vi "Load Obj File.vi"(5 "Load Material Textures (Default: True)":bool=TRUE, 6 "Material Search Folder (Default: <Not A Path> - Use Model Path Folder)":path=path "", 7 "Force Regenerate Normals (Defaut: False)":bool, 8 "error in (no error)":errorcluster, 11 "Object Model Path":path) -> (0 "error out":errorcluster, 3 "Objects":refnum<vi>[](array[refnum]), 4 "Bounding Box":T1)   [LabVIEW 2020, in "g_ar_toolkit.ar.lvlib"]
uses:
  g_ar_toolkit.ar.lvlib
  Model Bounding Box.ctl
  g_ar_toolkit.common/Object Point (Float).ctl
  Vertex Descriptor.ctl
  <vilib>/Utility/miscctls.llb/LV3DPointTypeDef.ctl
  <vilib>/picture/3D Picture Control/Geometries/Create Mesh.vi
  <vilib>/picture/3D Picture Control/Object/Create Object.vi
  <vilib>/picture/3D Picture Control/Object/Create Object (drawable).vi
  <vilib>/picture/3D Picture Control/Object/Set Material.vi
  <vilib>/Utility/libraryn.llb/Get File Extension.vi
  <vilib>/picture/jpeg.llb/Read JPEG File.vi
  <vilib>/picture/3D Picture Control/Helpers/Apply Texture.vi
  <vilib>/picture/3D Picture Control/Helpers/Apply Texture (no reference).vi
  <vilib>/picture/png.llb/Read PNG File.vi
  <vilib>/picture/bmp.llb/Read BMP File.vi
  bin/g_ar_toolkit.1.32.dll
  g_ar_toolkit.common/g_ar_toolkit.common.lvlib
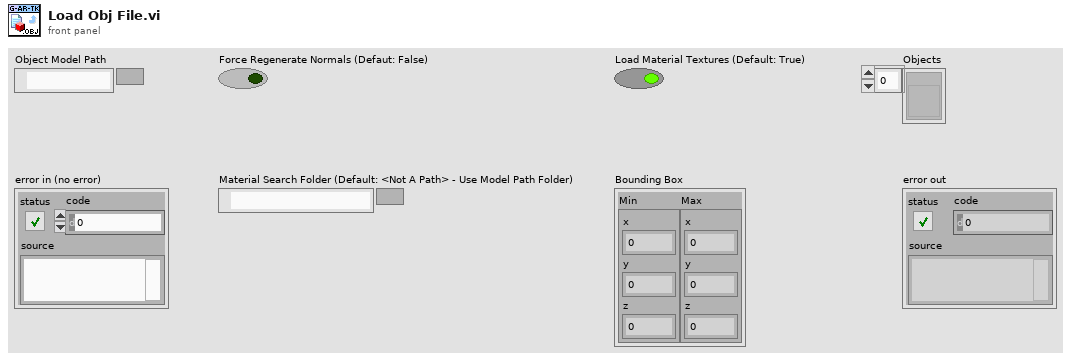
[diagram p1: front panel]
types:
  T1 = typedef "g_ar_toolkit.ar.lvlib/Model Bounding Box.ctl" = cluster{"Min":T2, "Max":T2}
  T2 = typedef "g_ar_toolkit.common.lvlib/Object Point (Float).ctl" = cluster{"x":dbl, "y":dbl, "z":dbl}
  T3 = typedef "g_ar_toolkit.ar.lvlib/Vertex Descriptor.ctl" = cluster{"Vertex":T4, "Normal":T4, "Colour":cluster{"R":sgl, "G":sgl, "B":sgl}, "Texture Coord":cluster{"S":sgl, "T":sgl}}
  T4 = typedef "LV3DPointTypeDef.ctl" = cluster{"X":sgl, "Y":sgl, "Z":sgl}
  T5 = cluster{"Name":string, "Shininess":sgl, "Ambient":cluster{"Red":sgl, "Green":sgl, "Blue":sgl}, "Specular":cluster{"Red":sgl, "Green":sgl, "Blue":sgl}, "Emission":cluster{"Red":sgl, "Green":sgl, "Blue":sgl}, "Diffuse":cluster{"Red":sgl, "Green":sgl, "Blue":sgl}, "texture-name":string}[]
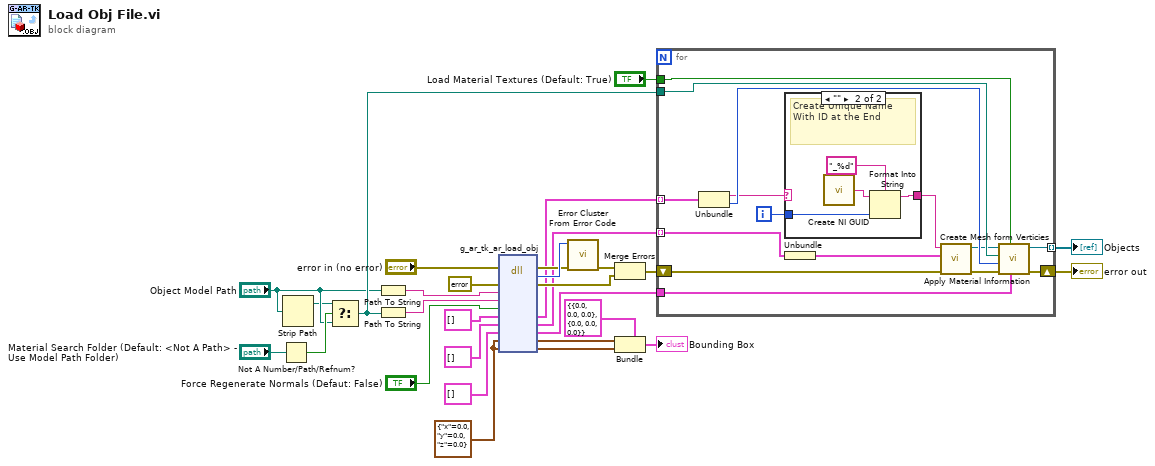
[diagram p0: block diagram]
diagram:
  w20 = T2 {"x"=0.0, "y"=0.0, "z"=0.0} ("Object Point")
  n1 = Not A Number/Path/Refnum?(number/path/refnum="Material Search Folder (Default: <Not A Path> - Use Model Path Folder)") -> (NaN/Path/Refnum?=w4:bool)
  n2 = Strip Path(path="Object Model Path") -> (stripped path=w1:path)  [unwired: 1 out]
  n3 = Select(t=w1, s=w4, f="Object Model Path") -> (s? t:f=w3:path)
  n4 = Path To String(path="Object Model Path") -> (string=w19:string)
  n5 = Path To String(path=w3) -> (string=w18:string)
  n6 = dll-call lib="C:/serenial/libraries/g-augmented-reality-toolkit/LabVIEW/bin/g_ar_toolkit.1.*.*" fn="g_ar_tk_ar_load_obj" ("g_ar_toolkit.*.*:g_ar_tk_image_copy")(error in="error in (no error)", "error_cluster"=errorcluster {"status"=FALSE, "code"=0, "source"=""} ("error constant"), "object_path"=w19, "material_path"=w18, "regen_normals"="Force Regenerate Normals (Defaut: False)", "object_array"=cluster{"name":string, "material_id":i32}[] [], "point_arrays"=cluster{"Verticies":T3[]}[] [], "material_array"=T5 [] ("Materials"), "bbox_min"=w20, "bbox_max"=w20) -> (error out=w24:errorcluster, "MgErr"=w25:i32, "error_cluster"=w28:errorcluster, "object_array"=w15:cluster{"name":string, "material_id":i32}[], "point_arrays"=w11:cluster{"Verticies":T3[]}[], "material_array"=w10:T5, "bbox_min"=w8:T2, "bbox_max"=w7:T2)  [unwired: 5 in, 1 out]
  n7 = call <vilib>:"Error Cluster From Error Code.vi"("error in (no error)"=w24, "error code (0)"=w25) -> ("error out"=w26:errorcluster)  [unwired: 7 in]
  n8 = Merge Errors(w26, w28) -> (w16:errorcluster)
  n9 = Bundle(cluster=T1 {"Min"={"x"=0.0, "y"=0.0, "z"=0.0}, "Max"={"x"=0.0, "y"=0.0, "z"=0.0}} ("Bounding Box"), "Min"=w8, "Max"=w7) -> (→"Bounding Box":T1)
  n10 = for {
    tunnel: w15 -> [w44] mode=indexing
    tunnel: [w43] -> w14 mode=indexing
    tunnel: w10 -> [w41]
    shift-right: [w42] -> w13
    shift-left: w16 -> [w40]
    tunnel: w3 -> [w38]
    tunnel: w11 -> [w34] mode=indexing
    tunnel: "Load Material Textures (Default: True)" -> [w30]
    i -> [w36]
    n11 = Unbundle(w44) -> ("name"=w37:string, "material_id"=w39:i32)
    n12 = case shown="\"\"" w37 {
      selector: w37 -> [w45 _]
      tunnel: w36 -> [_ w49]
      tunnel: [w45 w46] -> w35
      frame Default {
      }
      frame "" {
        # "Create Unique Name With ID at the End"
        n13 = call <vilib>:"Create NI GUID.vi"() -> ("NI GUID"=w48:string)
        n14 = Format Into String(format string="_%d", initial string=w48, w49) -> (resulting string=w46:string)  [unwired: 1 in, 1 out]
      }
    }
    n15 = Unbundle(w34) -> ("Verticies"=w33:T3[])
    n16 = call "Create Mesh form Verticies.vi"("error in (no error)"=w40, "Verticies"=w33, "Object Name"=w35) -> ("error out"=w31:errorcluster, "SceneObject out"=w32:refnum<vi>)  [unwired: 7 in]
    n17 = call "Apply Material Information.vi"("Materials"=w41, "Load Material Textures"=w30, "error in (no error)"=w31, "material_id"=w39, "Material Path"=w38, "SceneObject in"=w32) -> ("error out"=w42:errorcluster, "SceneObject out"=w43:refnum<vi>)  [unwired: 4 in]
  }
  "Objects" <- w14
  "error out" <- w13
